vi "Receive RX Message.vi"(8 "error in (no error)":errorcluster, 11 "RxTx in":refnum<class "RxTx.lvclass">) -> (0 "error out":errorcluster, 3 "RxTx out":refnum<class "RxTx.lvclass">)   [LabVIEW 2018, in "RxTx.lvclass"]
uses:
  RxTx.lvclass
  RxTx.lvclass/RxTx.ctl
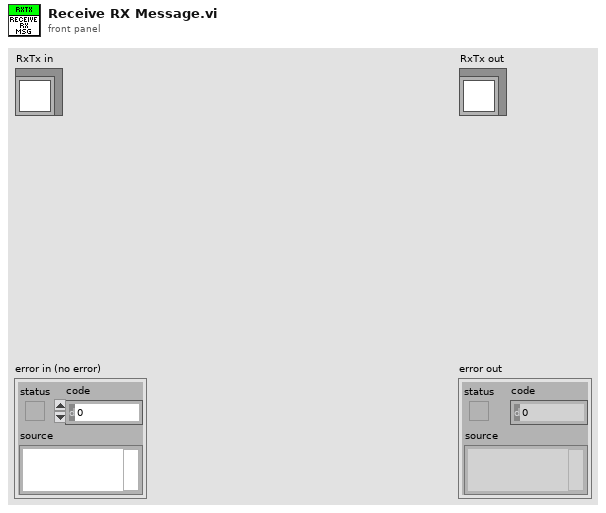
[diagram p1: front panel]
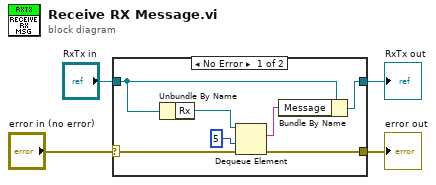
[diagram p0: block diagram]
diagram:
  n1 = case shown="No Error" "error in (no error)" {
    selector: "error in (no error)" -> [w9 w13]
    tunnel: [w10 w13] -> w3
    tunnel: [w6 w12] -> w1
    tunnel: "RxTx in" -> [w7 w12]
    frame No Error {
      n2 = Unbundle By Name(w7) -> ("Rx"=w11:refnum<queue>)
      n3 = Dequeue Element(queue=w11, timeout in ms (-1)=5, error in (no error)=w9) -> (element=w5:string, error out=w10:errorcluster)  [unwired: 2 out]
      n4 = Bundle By Name(cluster=w7, "Message"=w5) -> (w6:refnum<class "RxTx.lvclass">)
    }
    frame Error {
    }
  }
  "error out" <- w3
  "RxTx out" <- w1
